vi "test_generic.vi"() -> ()   [LabVIEW 2017, in "GenericStage.lvclass"]
uses:
  GenericStage.lvclass
  main/labview_source/type_definitions/clusters/controls_refs.ctl
  common/classes/SpaceVector/SpaceVector/SpaceVector.lvclass
  translation_mode_enum.ctl
  common/classes/GenericComponent/GenericComponent/GenericComponent.lvclass
  common/classes/ErrorController/ErrorController/ErrorController.lvclass
  common/classes/GenericToplevelComponent/GenericToplevelComponent/common_trigger_enum.ctl
  common/classes/GenericToplevelComponent/GenericToplevelComponent/GenericToplevelComponent.lvclass
panel:
  out "error loaded?":bool
  in  "createButton":bool
  in  "move relative":bool
  in  "move":bool
  in  "y":dbl[unit]
  in  "z":dbl[unit]
  in  "x":dbl[unit]
  in  "stop":bool
  # "Stage test"
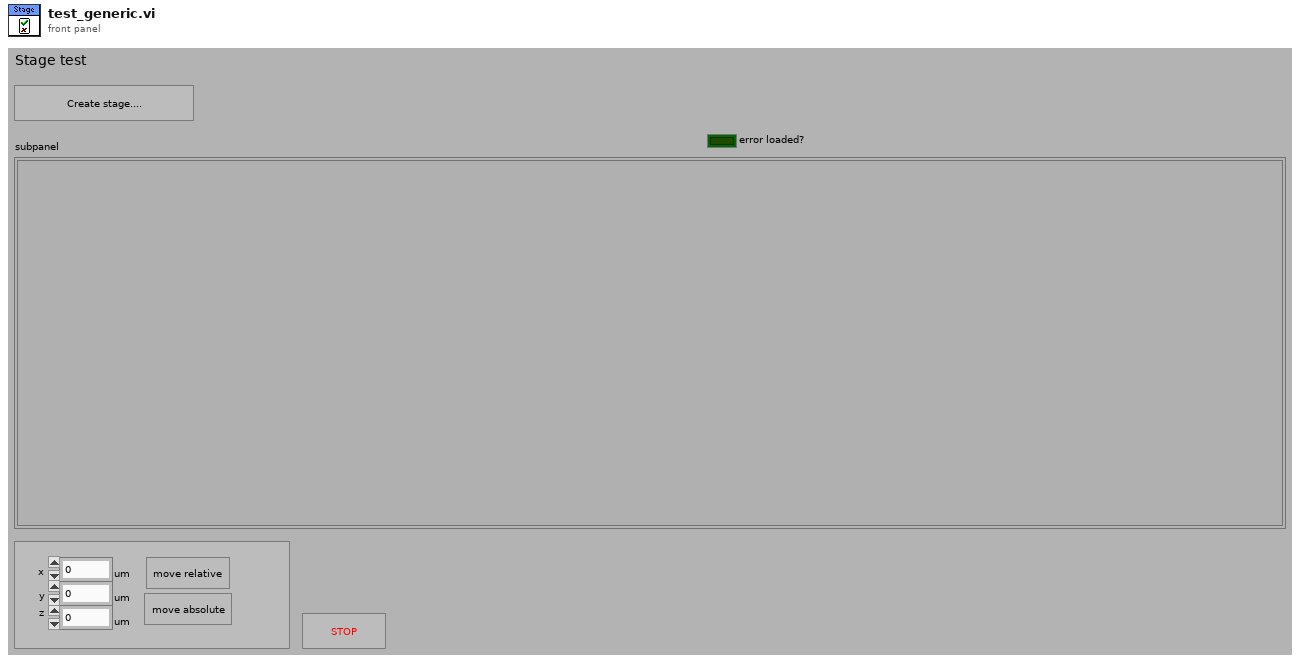
[diagram p1: front panel]
types:
  T1 = typedef "controls_refs.ctl" = cluster{"buttons":cluster{"start_focus":refnum<vi>, "start_single_sweep":refnum<vi>, "start_experiment":refnum<vi>, "save":refnum<vi>, "exit":refnum<vi>}, "tabs":cluster{"main":refnum<vi>, "settings":refnum<vi>}, "subpanels":cluster{"imagingMode":refnum<vi>, "scanHead":refnum<vi>, "display":refnum<vi>, "experimentController":refnum<vi>, "instrument":refnum<vi>, "stage":refnum<vi>, "stimulator":refnum<vi>, "dataCollection":refnum<vi>, "analyser":refnum<vi>, "daq":refnum<vi>, "imageAssembler":refnum<vi>}, "drop-downs":cluster{"imagingMode":refnum<vi>, "experimentalController":refnum<vi>, "objective":refnum<vi>}, "status lights":cluster{"experimentController":refnum<vi>, "imagingMode":refnum<vi>, "scanHead":refnum<vi>, "daq":refnum<vi>, "imageAssembler":refnum<vi>, "dataCollection":refnum<vi>, "display":refnum<vi>, "analyser":refnum<vi>, "stage":refnum<vi>, "stimulator":refnum<vi>, "instrument":refnum<vi>}, "message":refnum<vi>, "stimulator enabled?":refnum<vi>, "saving":cluster{"data folder path":refnum<vi>, "file base name":refnum<vi>, "notebook":refnum<vi>}, "progress bar":refnum<vi>, "update icon":refnum<vi>, "title":refnum<vi>, "main vi":refnum<vi>, "user":refnum<vi>}
  T2 = typedef "GenericStage.lvclass/translation_mode_enum.ctl" = enum16{"DON'T MOVE", "relative", "absolute"}
  T3 = typedef "GenericToplevelComponent.lvclass/common_trigger_enum.ctl" = enum16{"NULL", "initialise", "terminate", "fetch command", "fetch data", "attach observer", "register as observer", "detach observer", "acknowledge", "start", "stop", "sweep started", "sweep finished", "experiment started", "experiment stopped"}
  T4 = typedef "XComponentSpecification.xctl/data.ctl" = cluster{"class path":string, "configuration":string, "label":string, "settings name":string}
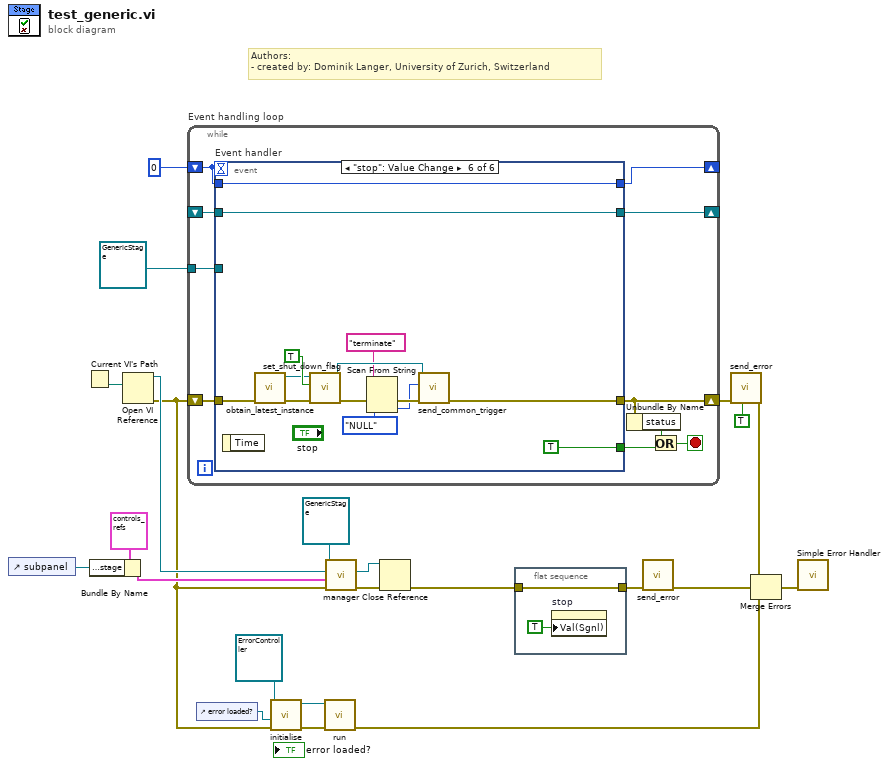
[diagram p0: block diagram]
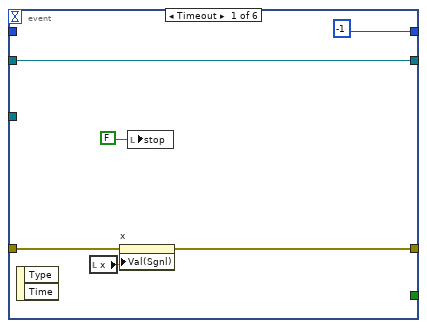
[diagram p2: hidden frame]
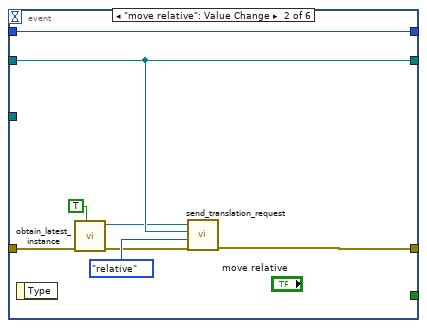
[diagram p3: hidden frame]
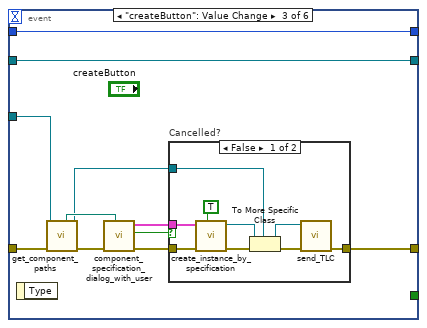
[diagram p4: hidden frame]
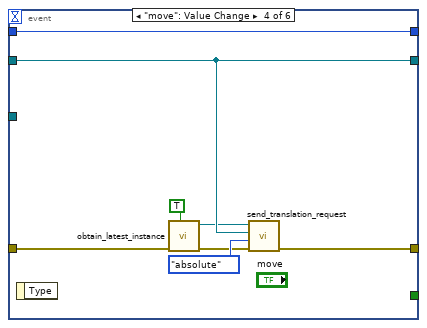
[diagram p6: hidden frame]
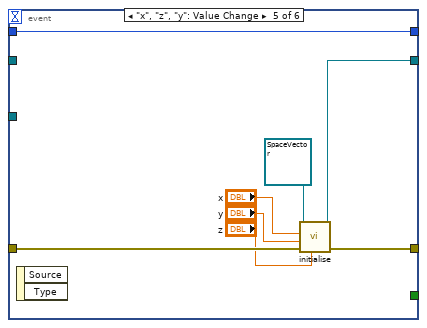
[diagram p7: hidden frame]
diagram:
  # "Authors: \n- created by: Dominik Langer, University of Zurich, Switzerland"
  n1 = control-ref of="subpanel"() -> (w22:refnum<vi>)
  n2 = Current VI's Path() -> (path=w19:path)
  n3 = Bundle By Name(cluster=T1 {"buttons"={"start_focus"=refnum, "start_single_sweep"=refnum, "start_experiment"=refnum, "save"=refnum, "exit"=refnum}, "tabs"={"main"=refnum, "settings"=refnum}, "subpanels"={"imagingMode"=refnum, "scanHead"=refnum, "display"=refnum, "experimentController"=refnum, "instrument"=refnum, "stage"=refnum, "stimulator"=refnum, "dataCollection"=refnum, "analyser"=refnum, "daq"=refnum, "imageAssembler"=refnum}, "drop-downs"={"imagingMode"=refnum, "experimentalController"=refnum, "objective"=refnum}, "status lights"={"experimentController"=refnum, "imagingMode"=refnum, "scanHead"=refnum, "daq"=refnum, "imageAssembler"=refnum, "dataCollection"=refnum, "display"=refnum, "analyser"=refnum, "stage"=refnum, "stimulator"=refnum, "instrument"=refnum}, "message"=refnum, "stimulator enabled?"=refnum, "saving"={"data folder path"=refnum, "file base name"=refnum, "notebook"=refnum}, "progress bar"=refnum, "update icon"=refnum, "title"=refnum, "main vi"=refnum, "user"=refnum} ("control references"), "subpanels.stage"=w22) -> (w21:T1)
  n4 = Open VI Reference(vi path=w19) -> (vi reference=w18:refnum<vi>, error out=w10:errorcluster)  [unwired: 5 in]
  n5 = while "Event handling loop" {
    shift-right: [w24] -> w7
    shift-left: w10 -> [w33]
    shift-right: [w31] -> _
    shift-left: 0 -> [w32]
    shift-right: [w30] -> _
    shift-left: _ -> [w29]
    tunnel: refnum<class "GenericStage.lvclass"> refnum ("GenericStage.lvclass") -> [w28]
    stop <- w25 stop-if-true
    n6 = event "Event handler" shown="[5] \"stop\": Value Change" {
      selector: _ -> [_ _ _ _ _ _]
      dyn-events: _ -> [_ _ _ _ _ _]
      timeout: w32 -> [_ _ _ _ _ _]
      tunnel: [_ _ _ _ _ TRUE] -> w26
      tunnel: w33 -> [w35 w43 w53 w72 w83 w88]
      tunnel: w32 -> [_ w47 w58 w76 w84 w97]
      tunnel: [-1 w47 w58 w76 w84 w97] -> w31
      tunnel: [w34 w46 w56 w75 w82 w85] -> w24
      tunnel: [w37 w44 w57 w74 w78 w96] -> w30
      tunnel: w29 -> [w37 w44 w57 w74 _ w96]
      tunnel: w28 -> [_ _ w50 _ _ _]
      event Timeout {
        n7 = event-data() -> ()  [unwired: 3 out]
        n8 = local read "x"() -> (w36:dbl[unit])
        n9 = property on="x" class="DigNum (strict)"(error in=w35, "Val(Sgnl)"=w36) -> (error out=w34:errorcluster)  [unwired: 1 in, 1 out]
        n10 = local write "stop"(FALSE) -> ()
      }
      event "move relative": Value Change {
        n11 = event-data() -> ()  [unwired: 2 out]
        n12 = call "obtain_latest_instance.vi"("quick, but maybe outdated?"=TRUE, "error in (no error)"=w43) -> ("error out"=w42:errorcluster, "GenericStage out"=w41:refnum<class "GenericStage.lvclass">)  [unwired: 8 in]
        n13 = call-dynamic "send_translation_request.vi"("error in (no error)"=w42, "translation mode"=translation_mode_enum."relative", "translation vector"=w44, "GenericStage in"=w41) -> ("error out"=w46:errorcluster)  [unwired: 7 out]
      }
      event "createButton": Value Change {
        n14 = event-data() -> ()  [unwired: 2 out]
        n15 = call-dynamic "get_component_paths.vi"("error in (no error)"=w53, "GenericComponent in"=w50) -> ("error out"=w54:errorcluster, "GenericComponent out"=w49:refnum<class "GenericStage.lvclass">, "component type directory"=w55:path)  [unwired: 4 in, 3 out]
        n16 = call "component_specification_dialog_with_user.vi"("start path"=w55, "error in (no error)"=w54) -> ("error out"=w52:errorcluster, "cancelled?"=w48:bool, "component specification out"=w51:T4)  [unwired: 7 in]
        n17 = case "Cancelled?" shown="False" w48 {
          tunnel: [w64 w68] -> w56
          tunnel: w52 -> [w61 w68]
          tunnel: w51 -> [w60 _]
          tunnel: w49 -> [w59 _]
          frame False {
            n18 = call "create_instance_by_specification.vi"("call constructor?"=TRUE, "error in (no error)"=w61, "component specification"=w60) -> ("error out"=w67:errorcluster, "GenericPlugin out"=w66:refnum<class "GenericComponent.lvclass">)  [unwired: 6 in, 1 out]
            n19 = To More Specific Class(target class=w59, reference=w66, error in=w67) -> (specific class reference=w63:refnum<class "GenericStage.lvclass">, error out=w65:errorcluster)
            n20 = call-dynamic "send_TLC.vi"("error in (no error)"=w65, "GenericToplevelComponent in"=w63) -> ("error out"=w64:errorcluster)  [unwired: 8 in, 1 out]
          }
          frame True {
          }
        }
      }
      event "move": Value Change {
        n21 = event-data() -> ()  [unwired: 2 out]
        n22 = call "obtain_latest_instance.vi"("quick, but maybe outdated?"=TRUE, "error in (no error)"=w72) -> ("error out"=w71:errorcluster, "GenericStage out"=w69:refnum<class "GenericStage.lvclass">)  [unwired: 8 in]
        n23 = call-dynamic "send_translation_request.vi"("error in (no error)"=w71, "translation mode"=translation_mode_enum."absolute", "translation vector"=w74, "GenericStage in"=w69) -> ("error out"=w75:errorcluster)  [unwired: 7 out]
      }
      event "x", "z", "y": Value Change {
        n24 = event-data() -> ()  [unwired: 3 out]
        n25 = call "initialise.vi"("z"="z", "error in (no error)"=w83, "y"="y", "x"="x", "SpaceVector in"=refnum<class "SpaceVector.lvclass"> refnum) -> ("error out"=w82:errorcluster, "SpaceVector out"=w78:refnum<class "SpaceVector.lvclass">)  [unwired: 5 out]
      }
      event "stop": Value Change {
        n26 = event-data() -> ()  [unwired: 2 out]
        n27 = call "obtain_latest_instance.vi"("error in (no error)"=w88) -> ("error out"=w87:errorcluster, "GenericStage out"=w86:refnum<class "GenericStage.lvclass">)  [unwired: 9 in]
        n28 = call-dynamic "set_shut_down_flag.vi"("error in (no error)"=w87, "shut down?"=TRUE, "GenericPlugin in"=w86) -> ("error out"=w92:errorcluster, "GenericPlugin out"=w94:refnum<class "GenericStage.lvclass">)  [unwired: 7 in]
        n29 = Scan From String(input string="terminate", error in=w92, default 1=common_trigger_enum."NULL" ("trigger")) -> (error out=w93:errorcluster, output 1=w89:T3)  [unwired: 2 in, 2 out]
        n30 = call-dynamic "send_common_trigger.vi"("error in (no error)"=w93, "trigger"=w89, "GenericToplevelComponent in"=w94) -> ("error out"=w85:errorcluster)  [unwired: 6 in, 2 out]
      }
    }
    n31 = Unbundle By Name(w24) -> ("status"=w27:bool)
    n32 = Or(x=w27, y=w26) -> (x .or. y?=w25:bool)
  }
  n33 = control-ref of="error loaded?"() -> (w12:refnum<vi>)
  n34 = call-dynamic "initialise.vi"("error in (no error)"=w10, "error boolean"=w12, "ErrorController in"=refnum<class "ErrorController.lvclass"> refnum ("ErrorController.lvclass")) -> ("error out"=w14:errorcluster, "ErrorController out"=w13:refnum<class "ErrorController.lvclass">)  [unwired: 7 in]
  n35 = call "run.vi"("error in (no error)"=w14, "ErrorController in"=w13) -> ("error out"=w9:errorcluster)  [unwired: 8 in, 1 out]
  n36 = call-dynamic "manager.vi"("error in (no error)"=w10, "control references"=w21, "top-level VI ref in"=w18, "GenericToplevelComponent in"=refnum<class "GenericStage.lvclass"> refnum ("GenericStage.lvclass")) -> ("error out"=w17:errorcluster, "top-level VI ref out"=w16:refnum<vi>)  [unwired: 5 in, 1 out]
  n37 = Close Reference(reference=w16, error in (no error)=w17) -> (error out=w4:errorcluster)
  n38 = flat-sequence {
    tunnel: [w100] -> w1
    tunnel: w4 -> [w100]
    frame #0 {
      n39 = property on="stop" class="Bool (strict)"("Val(Sgnl)"=TRUE ("Value (Signaling)")) -> ()  [unwired: 2 in, 2 out]
    }
  }
  n40 = call "send_error.vi"("error in (no error)"=w1) -> ("error out"=w2:errorcluster)  [unwired: 10 in]
  n41 = call "send_error.vi"("last error? (F)"=TRUE, "error in (no error)"=w7) -> ("error out"=w6:errorcluster)  [unwired: 9 in]
  n42 = Merge Errors(w6, w2, w9) -> (w15:errorcluster)
  n43 = call <vilib>:"Simple Error Handler.vi"("error in (no error)"=w15) -> ()  [unwired: 4 in, 5 out]
